vi "project3.vi"() -> ()   [LabVIEW 2020]
uses:
  <vilib>/vision/Image Controls.llb/IMAQ Image.ctl
panel:
  in  "Process":bool
  in  "Stop acquisition":bool
  in  "Acquire":bool
  out "Image":T1(plugin-control)
  in  "Stop program":bool
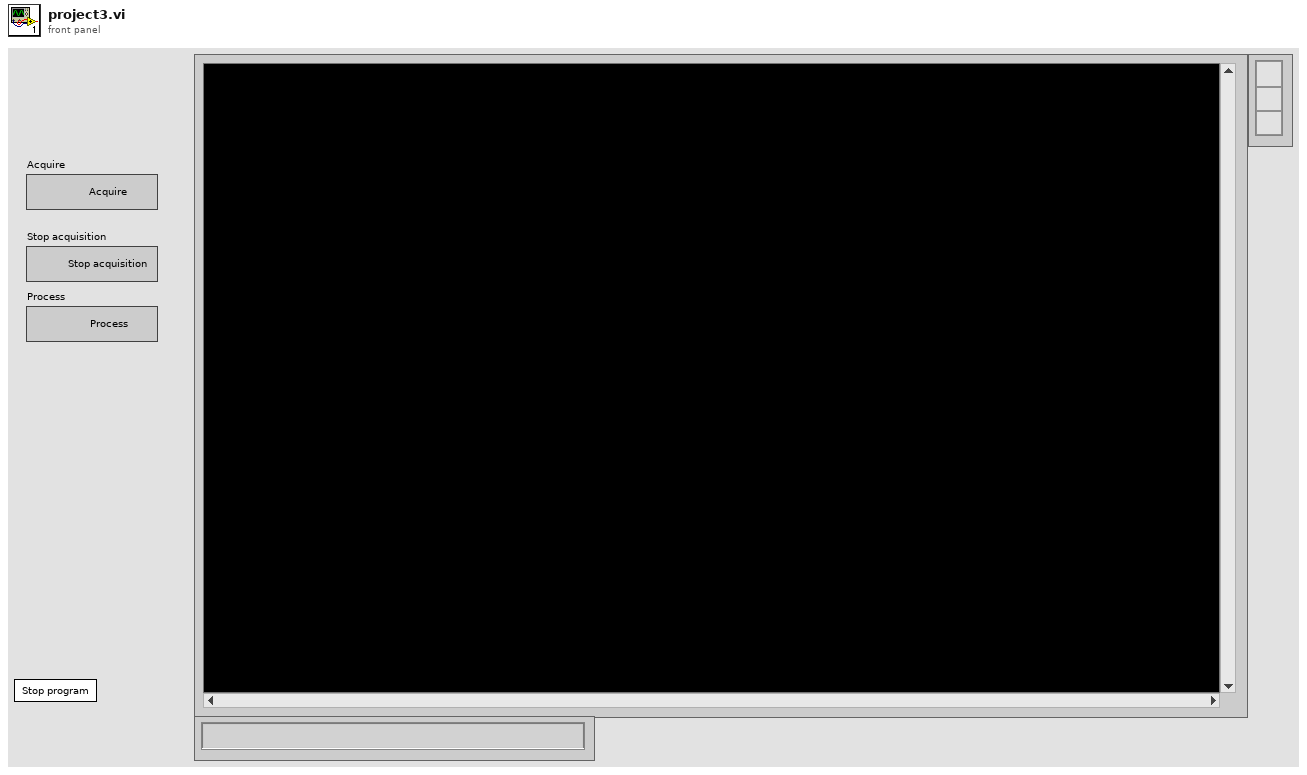
[diagram p1: front panel]
types:
  T1 = typedef "IMAQ Image.ctl" = refnum<image>
  T2 = enum32{"Invalid", "Standard", "Closed", "Hidden", "Minimized", "Maximized"}
  T3 = enum32{"invalid app kind", "Development System", "Run Time System", "Student Edition", "Embedded LabVIEW", "Evaluation", "Custom"}
  T4 = cluster{"Core":cluster{"Current VI Reference":refnum<vi>, "Close Panel on Exit?":bool}, "Aborted":bool, "New Image":T1, "Processing":bool}
  T5 = cluster{"Current VI Reference":refnum<vi>, "Close Panel on Exit?":bool}
  T6 = typedef "Image Type" = u32
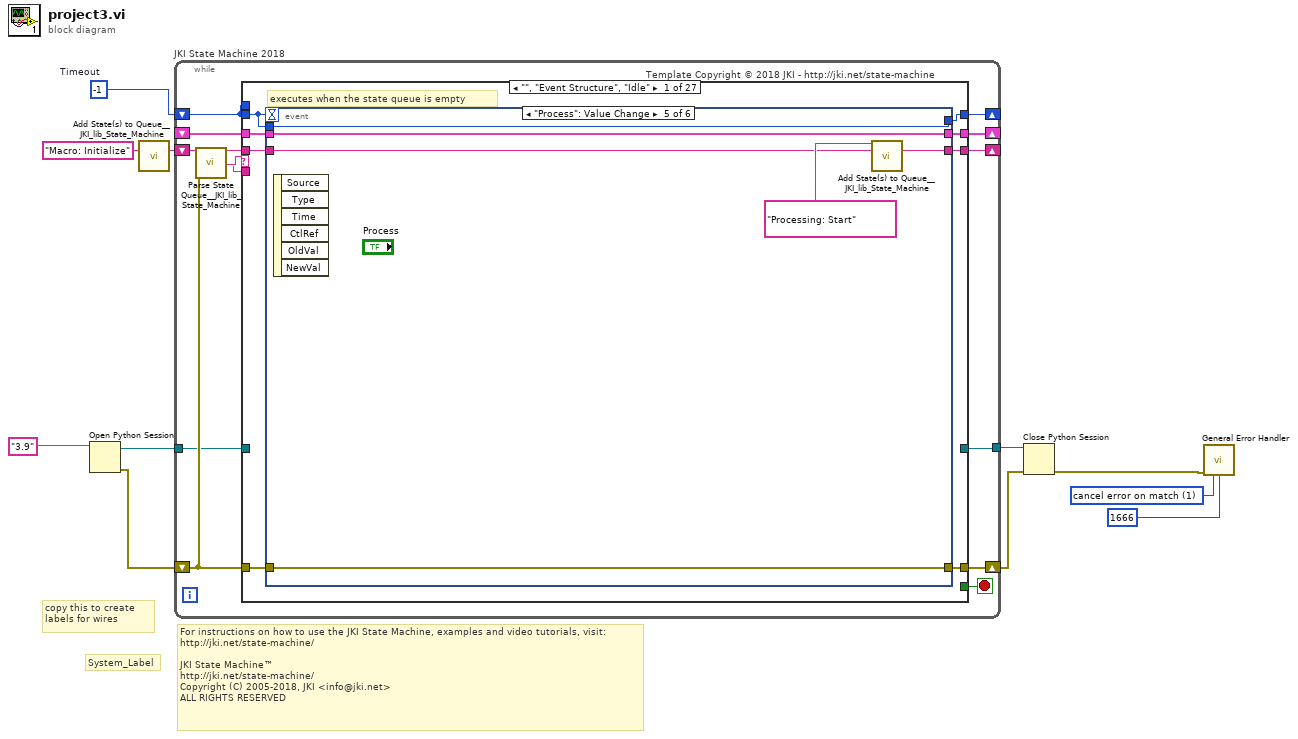
[diagram p0: block diagram]
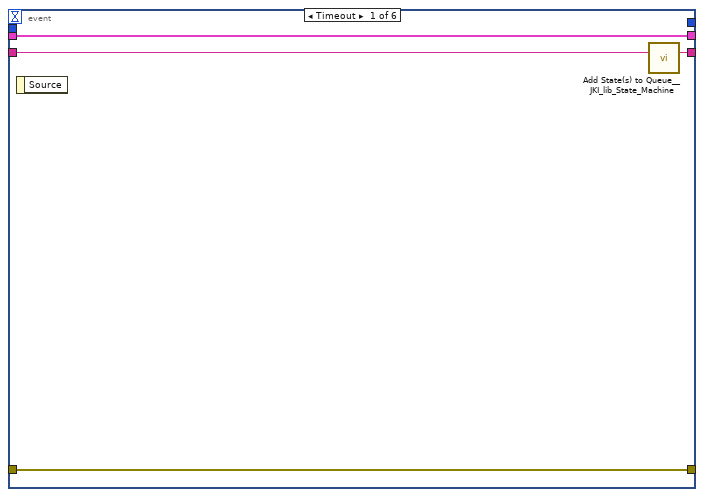
[diagram p2: hidden frame]
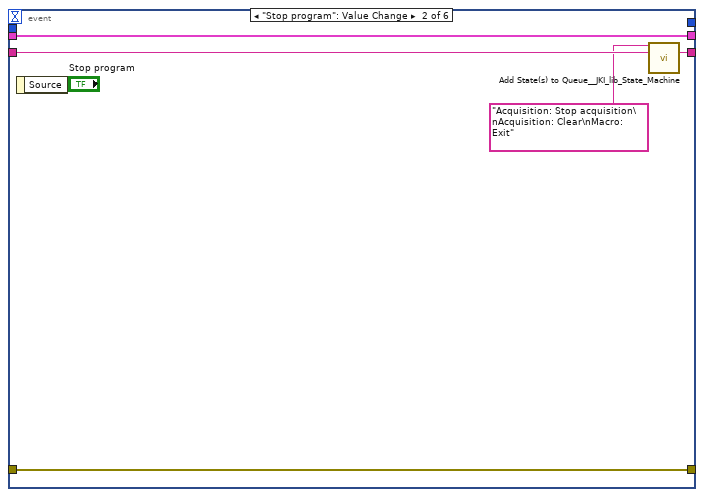
[diagram p3: hidden frame]
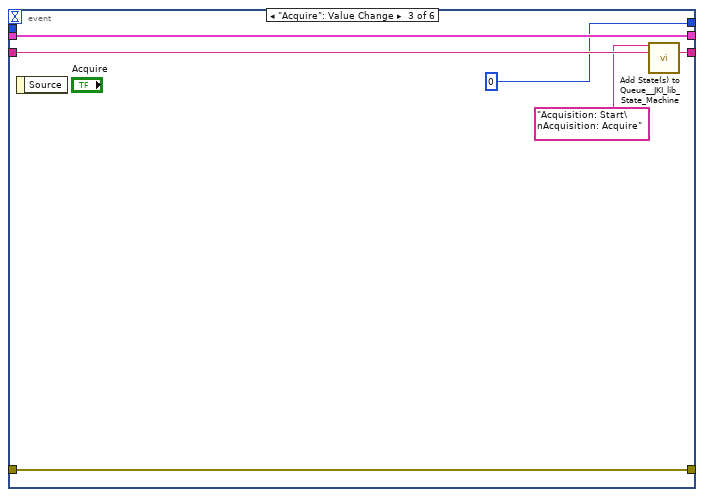
[diagram p4: hidden frame]
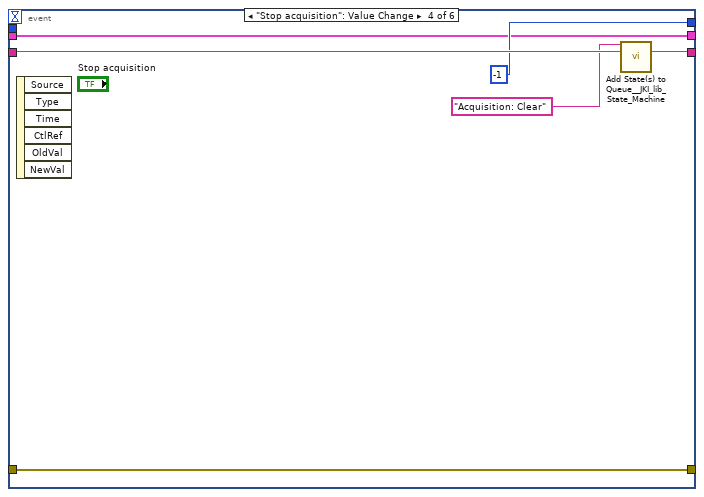
[diagram p5: hidden frame]
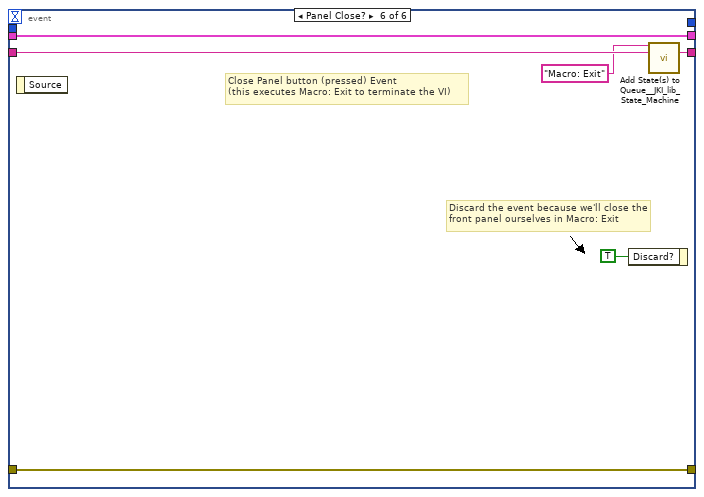
[diagram p6: hidden frame]
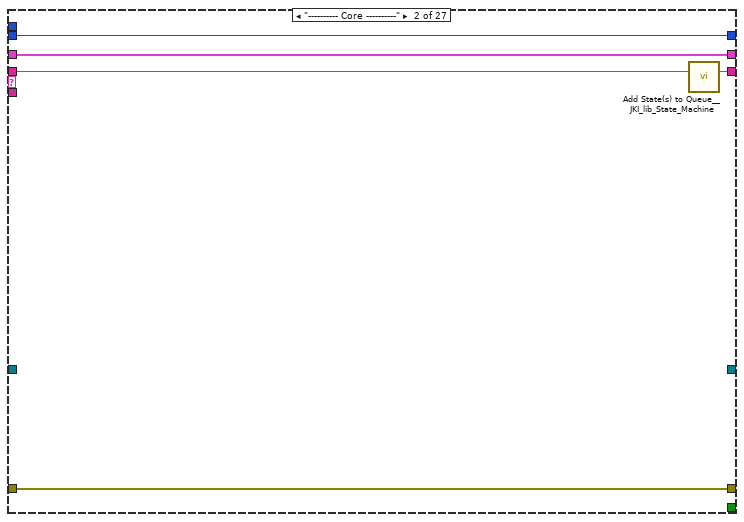
[diagram p7: hidden frame]
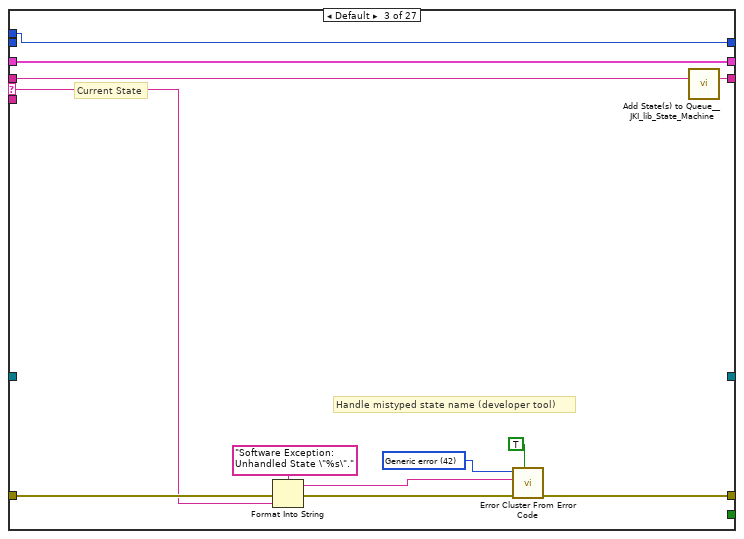
[diagram p8: hidden frame]
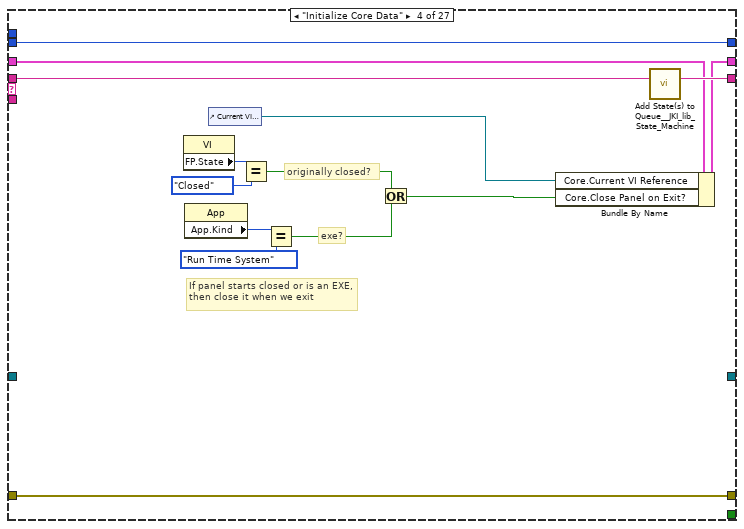
[diagram p9: hidden frame]
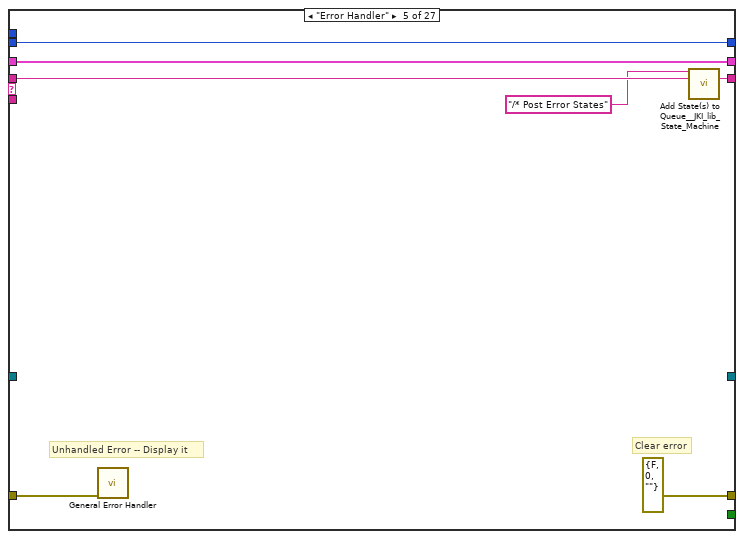
[diagram p10: hidden frame]
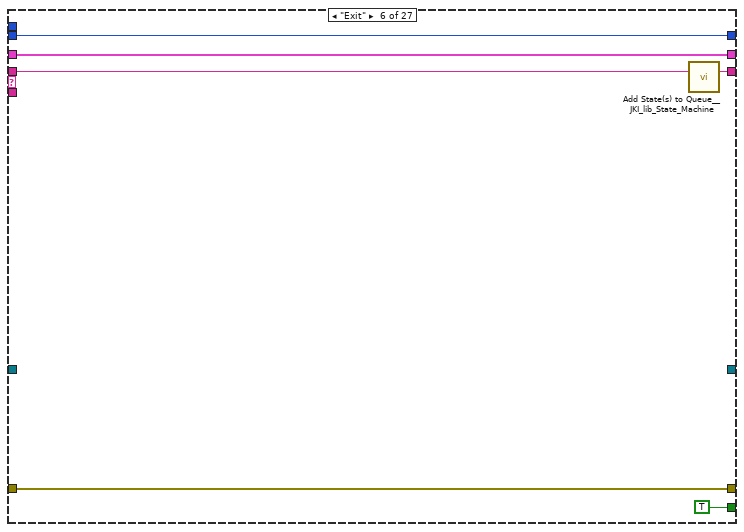
[diagram p11: hidden frame]
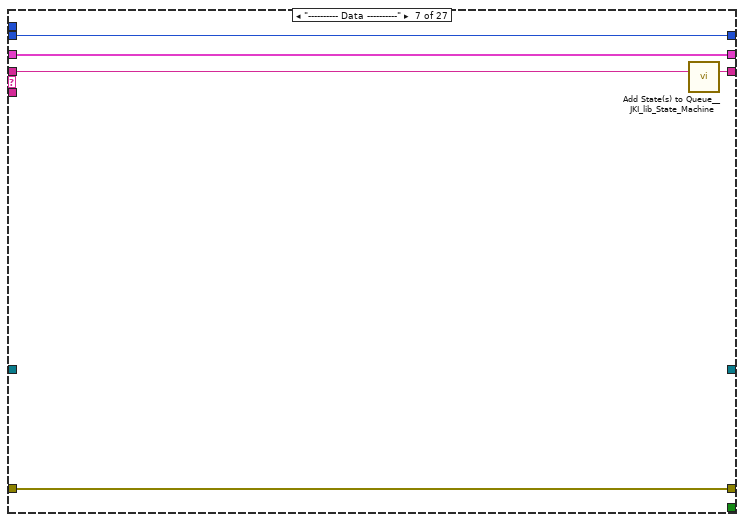
[diagram p12: hidden frame]
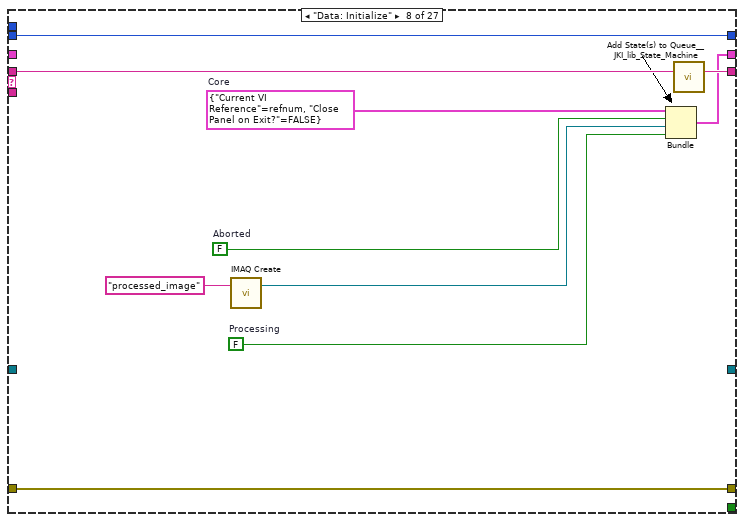
[diagram p13: hidden frame]
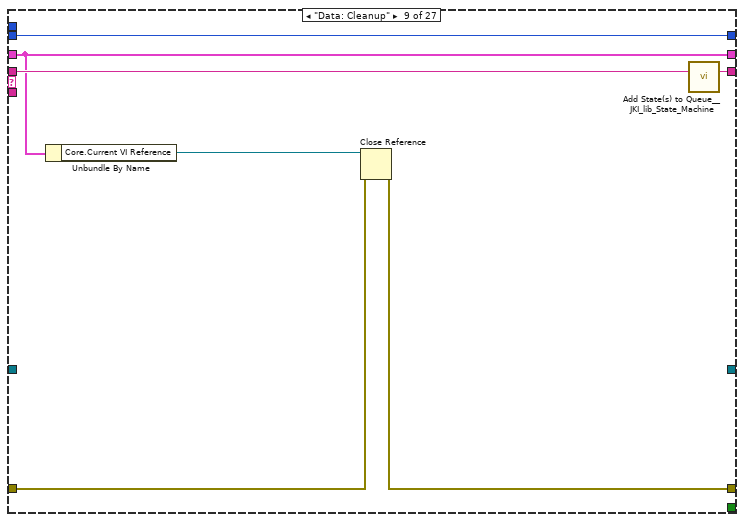
[diagram p14: hidden frame]
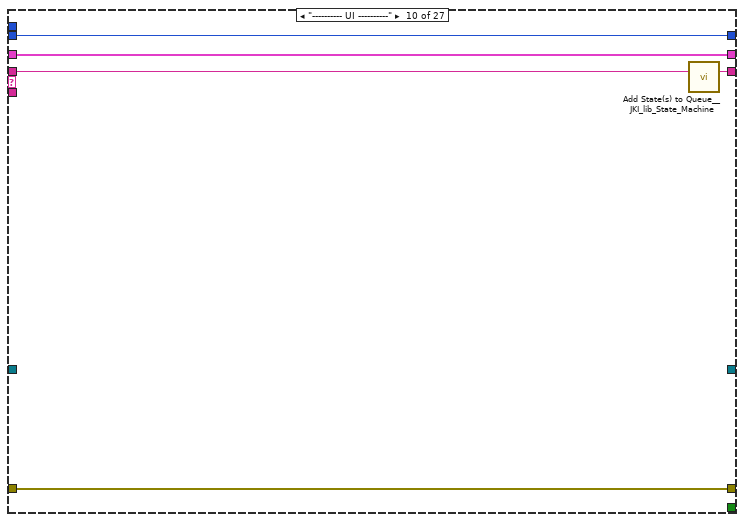
[diagram p15: hidden frame]
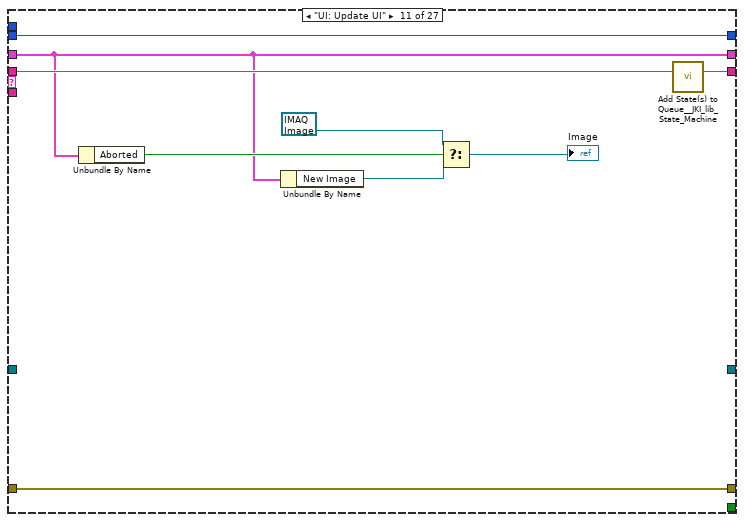
[diagram p16: hidden frame]
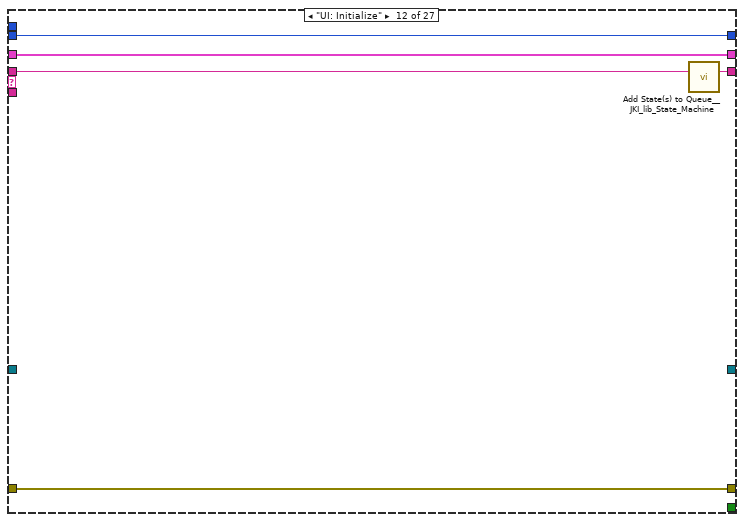
[diagram p17: hidden frame]
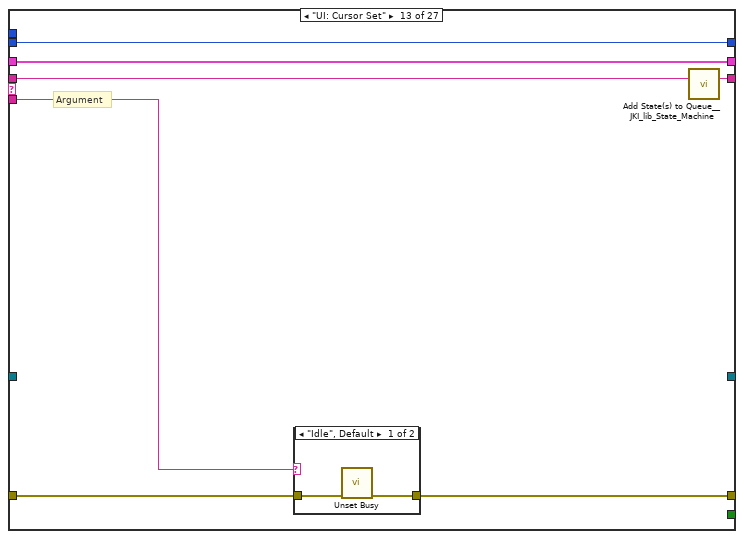
[diagram p18: hidden frame]
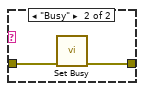
[diagram p19: hidden frame]
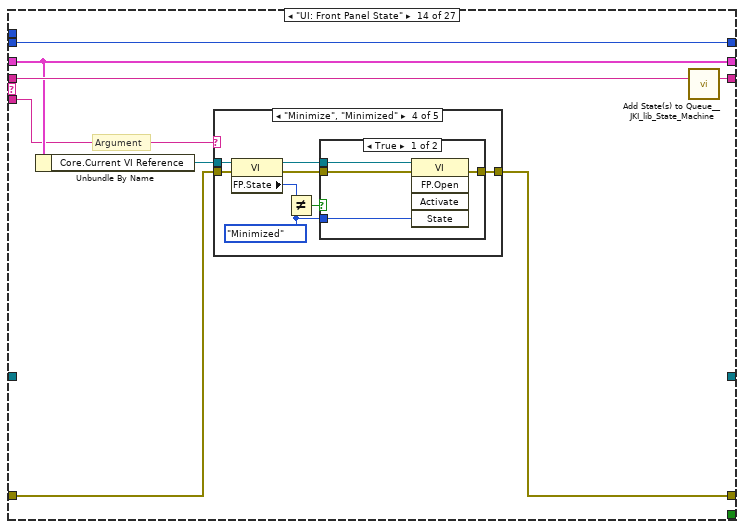
[diagram p20: hidden frame]
diagram:
  w3 = 1 items=["no exception", "cancel error on match", "set error on match"] ("[exception action] (none:0)")
  w9 = -1  # Timeout
  # "For instructions on how to use the JKI State Machine, examples and video tutorials, visit:\nhttp://jki.net/state-machine/\n\nJKI State Machine™\nhttp://jki.net/state-machine/\nCopyright (C) 2005-2018, JKI <info@jki.net>\nALL RIGHTS RESERVED"
  # "copy this to create labels for wires"
  # "System_Label"
  n1 = Open Python Session(python version="3.9" ("Python version")) -> (session out=w8:refnum<k35>, error out=w6:errorcluster)  [unwired: 2 in]
  n2 = call <vilib>:"Add State(s) to Queue__JKI_lib_State_Machine.vi"("State(s) in (\"\")"="Macro: Initialize") -> ("States Out"=w11:string)  [unwired: 14 in]
  n3 = while "JKI State Machine 2018" {
    shift-right: [w18] -> _
    shift-left: _ -> [w17]
    shift-right: [w21] -> w4
    shift-left: w6 -> [w16]
    shift-right: [w20] -> _
    shift-left: w11 -> [w22]
    shift-right: [w15] -> _
    shift-left: w9 -> [w14]
    tunnel: w8 -> [w13]
    tunnel: [w12] -> w5
    stop <- w19 stop-if-true
    # "Template Copyright © 2018 JKI - http://jki.net/state-machine"
    n4 = call <vilib>:"Parse State Queue__JKI_lib_State_Machine.vi"("State Queue"=w22, "Error In (no error)"=w16) -> ("Remaining States"=w24:string, "Current State"=w25:string, "Arguments"=w23:string)  [unwired: 11 in]
    n5 = case shown="\"\", \"Event Structure\", \"Idle\"" w25 {
      selector: w25 -> [_ _ w73 _ _ _ _ _ _ _ _ _ _ _ _ _ _ _ _ _ _ _ _ _ _ _ _]
      tunnel: w24 -> [w33 w71 w77 w97 w104 w110 w115 w125 w132 w137 w145 w151 w158 w170 w240 w246 w257 w262 w269 w286 w293 w302 w307 w312 w319 w339 w344]
      tunnel: w23 -> [_ _ _ _ _ _ _ _ _ _ _ _ w153 w164 _ _ _ _ _ _ _ _ _ _ _ _ _]
      tunnel: w17 -> [w31 w68 w75 w90 w101 w108 w112 _ w127 w134 w141 w149 w156 w166 w237 w243 w254 w259 w264 w284 w289 w298 w304 w309 w315 w335 w341]
      tunnel: [w30 w69 w79 w94 errorcluster {"status"=FALSE, "code"=0, "source"=""} ("error out") w107 w113 w122 w128 w135 w139 w148 w154 w167 w238 w244 w255 w260 w267 w274 w291 w300 w305 w310 w317 w328 w342] -> w21
      tunnel: w16 -> [w29 w69 w78 w94 w100 w107 w113 w122 w129 w135 w139 w148 w155 w168 w238 w244 w255 w260 w267 w275 w291 w300 w305 w310 w317 w327 w342]
      tunnel: [w32 w70 w76 w96 w103 w109 w114 w124 w131 w136 w146 w150 w157 w169 w239 w245 w256 w261 w268 w285 w292 w301 w306 w311 w318 w338 w343] -> w20
      tunnel: [_ _ _ _ _ TRUE _ _ _ _ _ _ _ _ _ _ _ _ _ _ _ _ _ _ _ _ _] -> w19
      tunnel: [w28 w68 w75 w95 w101 w108 w112 w123 w127 w134 w141 w149 w156 w166 w237 w243 w254 w259 w265 w283 w288 w298 w304 w309 w314 w334 w341] -> w18
      tunnel: w14 -> [w26 w67 _ w84 w98 w105 w111 w117 w126 w133 w138 w147 w152 w163 w236 w241 w247 w258 w263 w276 w290 w299 w303 w308 w316 w337 w340]
      tunnel: [w27 w67 w72 w84 w98 w105 w111 w117 w126 w133 w138 w147 w152 w163 w236 w241 w247 w258 w263 w276 w290 w299 w303 w308 w316 w337 w340] -> w15
      tunnel: w14 -> [_ _ w72 _ _ _ _ _ _ _ _ _ _ _ _ _ _ _ _ _ _ _ _ _ _ _ _]
      tunnel: w13 -> [_ _ _ _ _ _ _ _ _ _ _ _ _ _ _ _ _ _ _ _ _ _ _ _ _ w321 _]
      tunnel: [_ _ _ _ _ _ _ _ _ _ _ _ _ _ _ _ _ _ _ _ _ _ _ _ _ w320 _] -> w12
      frame "", "Event Structure", "Idle" {
        # "executes when the state queue is empty"
        n6 = event shown="[4] \"Process\": Value Change" {
          selector: _ -> [_ _ _ _ _ _]
          dyn-events: _ -> [_ _ _ _ _ _]
          timeout: w26 -> [_ _ _ _ _ _]
          tunnel: w33 -> [w37 w42 w48 w53 w55 w66]
          tunnel: [w36 w41 w47 w54 w59 w65] -> w32
          tunnel: w31 -> [w34 w39 w45 w50 w60 w63]
          tunnel: [w35 w40 w46 w49 w56 w64] -> w30
          tunnel: w29 -> [w35 w40 w46 w49 w56 w64]
          tunnel: [w34 w39 w45 w50 w60 w63] -> w28
          tunnel: [_ _ 0 ("Timeout") -1 ("Timeout") w57 _] -> w27
          tunnel: w26 -> [_ _ _ _ w57 _]
          event Timeout {
            n7 = event-data() -> ()  [unwired: 1 in, 1 out]
            n8 = call <vilib>:"Add State(s) to Queue__JKI_lib_State_Machine.vi"("State(s) in (\"\")"=w37) -> ("States Out"=w36:string)  [unwired: 14 in]
          }
          event "Stop program": Value Change {
            n9 = event-data() -> ()  [unwired: 1 in, 1 out]
            n10 = call <vilib>:"Add State(s) to Queue__JKI_lib_State_Machine.vi"("State(s) in Front (\"\")"="Acquisition: Stop acquisition\nAcquisition: Clear\nMacro: Exit", "State(s) in (\"\")"=w42) -> ("States Out"=w41:string)  [unwired: 13 in]
          }
          event "Acquire": Value Change {
            n11 = event-data() -> ()  [unwired: 1 in, 1 out]
            n12 = call <vilib>:"Add State(s) to Queue__JKI_lib_State_Machine.vi"("State(s) in Front (\"\")"="Acquisition: Start\nAcquisition: Acquire", "State(s) in (\"\")"=w48) -> ("States Out"=w47:string)  [unwired: 13 in]
          }
          event "Stop acquisition": Value Change {
            n13 = event-data() -> ()  [unwired: 1 in, 6 out]
            n14 = call <vilib>:"Add State(s) to Queue__JKI_lib_State_Machine.vi"("State(s) in Front (\"\")"="Acquisition: Clear" ("State(s) in Front (\"\")"), "State(s) in (\"\")"=w53) -> ("States Out"=w54:string)  [unwired: 13 in]
          }
          event "Process": Value Change {
            n15 = event-data() -> ()  [unwired: 1 in, 6 out]
            n16 = call <vilib>:"Add State(s) to Queue__JKI_lib_State_Machine.vi"("State(s) in Front (\"\")"="Processing: Start" ("State(s) in Front (\"\")"), "State(s) in (\"\")"=w55) -> ("States Out"=w59:string)  [unwired: 13 in]
          }
          event Panel Close? {
            # "Discard the event because we'll close the front panel ourselves in Macro: Exit"
            # "Close Panel button (pressed) Event\n(this executes Macro: Exit to terminate the VI)"
            n17 = event-data() -> ()  [unwired: 1 in, 1 out]
            n18 = event-data("Discard?"=TRUE) -> ()  [unwired: 1 in, 1 out]
            n19 = call <vilib>:"Add State(s) to Queue__JKI_lib_State_Machine.vi"("State(s) in Front (\"\")"="Macro: Exit", "State(s) in (\"\")"=w66) -> ("States Out"=w65:string)  [unwired: 13 in]
          }
        }
      }
      frame "---------- Core ----------" {
        n20 = call <vilib>:"Add State(s) to Queue__JKI_lib_State_Machine.vi"("State(s) in (\"\")"=w71) -> ("States Out"=w70:string)  [unwired: 14 in]
      }
      frame Default {
        w82 = 42 items=["No error", "Argument error", "Memory is full", "Out of zone", "End of file", "File already open", "Generic file I/O error", "File not found", "File permission error", "Disk is full", "Duplicate path", "Too many files open", "System feature not enabled", "Resource file not found", "Cannot add resource", "Resource not found", "Image not found", "Image memory error", "Pen does not exist", "Config type invalid", "Config token not found", "Config parse error", "Config memory error", "Bad external code format", "Bad external code offset", "External code not present", "Null window", "Destroy window error", "Null menu", "Print aborted", "Bad print record", "Print driver error", "Windows error during printing", "Memory error during printing", "Print dialog error", "Generic print error", "Invalid device refnum", "Device not found", "Device parameter error", "Device unit error", "Cannot open device", "Device call aborted", "Generic error", "Cancelled by user", "Object ID too low", "Object ID too high", "Object not in heap", "Unknown heap", "Unknown object (invalid DefProc)", "Unknown object (DefProc not in table)", "Message out of range", "Invalid (null) method", "Unknown message", "Manager call not supported", "Bad address", "Network operation in progress", "Network operation timed out", "Connection is busy", "Network attribute not supported", "Network error", "Address in use", "System out of memory", "Connection aborted", "Connection refused", "Not connected", "Already connected", "Connection closed", "Initialization error (interapplication manager)", "Bad occurrence", "Wait on unbound occurrence handler", "Occurrence queue overflow", "Datalog type conflict", "Unused", "Unrecognized type (interapplication manager)", "Memory corrupt", "Failed to make temporary DLL", "Old CIN version", "Drag socket not found", "Failed to load drop-object", "Failed to register OLE object", "Failed to release OLE object", "Format specifier type mismatch", "Unknown format specifier", "Too few format specifiers", "Too many format specifiers", "Scan failed", "Newer CIN version", "Error converting to variant", "Runtime menu error", "Password tampered", "Variant attribute not found", "Incompatible variant data type", "Event data is not available", "Event Store is not present", "Occurrence is not found", "Event Queue is not created", "Event info is not available", "Refnum passed is NULL", "Error retrieving Class GUID", "Error retrieving CoClass GUID", "Error retrieving TypeLib GUID.", "Bad built application magic bytes.", "Specific driver is different from the specific driver associated with the Logical Name.", "There is no session opened to the class driver.", "Max Error", "MAX - Error with config objects", "MAX - Error loading configuration", "MAX - Group not supported"]
        # "Current State"
        # "Handle mistyped state name (developer tool)"
        n21 = Format Into String(format string="Software Exception: Unhandled State \"%s\"." ("message"), error in=w78, w73) -> (resulting string=w81:string, error out=w80:errorcluster)  [unwired: 1 in]
        n22 = call <vilib>:"Error Cluster From Error Code.vi"("show call chain? (False)"=TRUE, "error in (no error)"=w80, "error message (\"\")"=w81, "error code (0)"=w82) -> ("error out"=w79:errorcluster)  [unwired: 5 in]
        n23 = call <vilib>:"Add State(s) to Queue__JKI_lib_State_Machine.vi"("State(s) in (\"\")"=w77) -> ("States Out"=w76:string)  [unwired: 14 in]
      }
      frame "Initialize Core Data" {
        # "originally closed?"
        # "exe?"
        # "If panel starts closed or is an EXE, then close it when we exit"
        n24 = property class="VI"() -> ("FP.State"=w87:T2)  [unwired: 2 in, 2 out]
        n25 = property class="App"() -> ("App.Kind"=w93:T3)  [unwired: 2 in, 2 out]
        n26 = control-ref of="Current VI Reference"() -> (w88:refnum<vi>)
        n27 = Equal?(x=w87, y=T2."Closed" ("Front Panel Window:State")) -> (x = y?=w85:bool)
        n28 = Equal?(x=w93, y=T3."Run Time System" ("Application:Kind")) -> (x = y?=w91:bool)
        n29 = Or(x=w85, y=w91) -> (x .or. y?=w89:bool)
        n30 = Bundle By Name(cluster=w90, "Core.Current VI Reference"=w88, "Core.Close Panel on Exit?"=w89) -> (w95:T4)
        n31 = call <vilib>:"Add State(s) to Queue__JKI_lib_State_Machine.vi"("State(s) in (\"\")"=w97) -> ("States Out"=w96:string)  [unwired: 14 in]
      }
      frame "Error Handler" {
        # "Unhandled Error -- Display it"
        # "Clear error"
        n32 = call <vilib>:"General Error Handler.vi"("error in (no error)"=w100) -> ()  [unwired: 10 in, 5 out]
        n33 = call <vilib>:"Add State(s) to Queue__JKI_lib_State_Machine.vi"("State(s) in Front (\"\")"="/* Post Error States", "State(s) in (\"\")"=w104) -> ("States Out"=w103:string)  [unwired: 13 in]
      }
      frame "Exit" {
        n34 = call <vilib>:"Add State(s) to Queue__JKI_lib_State_Machine.vi"("State(s) in (\"\")"=w110) -> ("States Out"=w109:string)  [unwired: 14 in]
      }
      frame "---------- Data ----------" {
        n35 = call <vilib>:"Add State(s) to Queue__JKI_lib_State_Machine.vi"("State(s) in (\"\")"=w115) -> ("States Out"=w114:string)  [unwired: 14 in]
      }
      frame "Data: Initialize" {
        w116 = FALSE  # Processing
        w120 = T5 {"Current VI Reference"=refnum, "Close Panel on Exit?"=FALSE}  # Core
        w121 = FALSE  # Aborted
        n36 = call "IMAQ Create"("Image Name"="processed_image") -> ("New Image"=w119:T1)  [unwired: 4 in, 1 out]
        n37 = Bundle("Core"=w120, "Aborted"=w121, "New Image"=w119, "Processing"=w116) -> (w123:T4)  [unwired: 1 in]
        n38 = call <vilib>:"Add State(s) to Queue__JKI_lib_State_Machine.vi"("State(s) in (\"\")"=w125) -> ("States Out"=w124:string)  [unwired: 14 in]
      }
      frame "Data: Cleanup" {
        n39 = Unbundle By Name(w127) -> ("Core.Current VI Reference"=w130:refnum<vi>)
        n40 = Close Reference(reference=w130, error in (no error)=w129) -> (error out=w128:errorcluster)
        n41 = call <vilib>:"Add State(s) to Queue__JKI_lib_State_Machine.vi"("State(s) in (\"\")"=w132) -> ("States Out"=w131:string)  [unwired: 14 in]
      }
      frame "---------- UI ----------" {
        n42 = call <vilib>:"Add State(s) to Queue__JKI_lib_State_Machine.vi"("State(s) in (\"\")"=w137) -> ("States Out"=w136:string)  [unwired: 14 in]
      }
      frame "UI: Update UI" {
        n43 = Unbundle By Name(w141) -> ("Aborted"=w144:bool)
        n44 = Unbundle By Name(w141) -> ("New Image"=w142:T1)
        n45 = Select(t=T1 refnum, s=w144, f=w142) -> (s? t:f=→"Image":T1)
        n46 = call <vilib>:"Add State(s) to Queue__JKI_lib_State_Machine.vi"("State(s) in (\"\")"=w145) -> ("States Out"=w146:string)  [unwired: 14 in]
      }
      frame "UI: Initialize" {
        n47 = call <vilib>:"Add State(s) to Queue__JKI_lib_State_Machine.vi"("State(s) in (\"\")"=w151) -> ("States Out"=w150:string)  [unwired: 14 in]
      }
      frame "UI: Cursor Set" {
        # "Argument"
        n48 = case shown="\"Idle\", Default" w153 {
          tunnel: w155 -> [w160 w162]
          tunnel: [w159 w161] -> w154
          frame "Idle", Default {
            n49 = call <vilib>:"Unset Busy.vi"("error in (no error)"=w160) -> ("error out"=w159:errorcluster)  [unwired: 10 in]
          }
          frame "Busy" {
            n50 = call <vilib>:"Set Busy.vi"("error in (no error)"=w162) -> ("error out"=w161:errorcluster)  [unwired: 9 in, 1 out]
          }
        }
        n51 = call <vilib>:"Add State(s) to Queue__JKI_lib_State_Machine.vi"("State(s) in (\"\")"=w158) -> ("States Out"=w157:string)  [unwired: 14 in]
      }
      frame "UI: Front Panel State" {
        # "Argument"
        n52 = Unbundle By Name(w166) -> ("Core.Current VI Reference"=w165:refnum<vi>)
        n53 = case shown="\"Minimize\", \"Minimized\"" w164 {
          tunnel: w168 -> [w176 w191 w202 w215 w228]
          tunnel: [w178 w192 w204 w217 w230] -> w167
          tunnel: w165 -> [w177 w189 w203 w216 w229]
          frame "Open", "Standard", Default {
            w171 = T2."Standard" ("State")
            n54 = property class="VI"(reference=w177, error in=w176) -> (reference out=w174:refnum<vi>, error out=w175:errorcluster, "FP.State"=w173:T2)
            n55 = Not Equal?(x=w173, y=w171) -> (x != y?=w172:bool)
            n56 = case shown="True" w172 {
              tunnel: [w182 w184] -> w178
              tunnel: w175 -> [w181 w184]
              tunnel: w174 -> [w180 _]
              tunnel: w171 -> [w179 _]
              frame True {
                n57 = invoke class="VI" method="FP.Open"(reference=w180, error in=w181, "Activate"=TRUE, "State"=w179) -> (error out=w182:errorcluster)  [unwired: 1 in, 4 out]
              }
              frame False {
              }
            }
          }
          frame "Close", "Closed" {
            n58 = property class="VI"(reference=w189, error in=w191) -> (reference out=w188:refnum<vi>, error out=w190:errorcluster, "FP.State"=w186:T2)
            n59 = Not Equal?(x=w186, y=T2."Closed" ("Front Panel Window:State")) -> (x != y?=w185:bool)
            n60 = case shown="True" w185 {
              tunnel: [w193 w196] -> w192
              tunnel: w190 -> [w193 w195]
              tunnel: w188 -> [_ w194]
              frame False {
              }
              frame True {
                n61 = invoke class="VI" method="FP.Close"(reference=w194, error in=w195) -> (error out=w196:errorcluster)  [unwired: 1 in, 2 out]
              }
            }
          }
          frame "Hidden", "Hide" {
            w197 = T2."Hidden" ("State")
            n62 = property class="VI"(reference=w203, error in=w202) -> (reference out=w200:refnum<vi>, error out=w201:errorcluster, "FP.State"=w199:T2)
            n63 = Not Equal?(x=w199, y=w197) -> (x != y?=w198:bool)
            n64 = case shown="True" w198 {
              tunnel: [w208 w209] -> w204
              tunnel: w201 -> [w207 w209]
              tunnel: w200 -> [w206 _]
              tunnel: w197 -> [w205 _]
              frame True {
                n65 = invoke class="VI" method="FP.Open"(reference=w206, error in=w207, "State"=w205) -> (error out=w208:errorcluster)  [unwired: 2 in, 4 out]
              }
              frame False {
              }
            }
          }
          frame "Minimize", "Minimized" {
            w210 = T2."Minimized" ("State")
            n66 = property class="VI"(reference=w216, error in=w215) -> (reference out=w213:refnum<vi>, error out=w214:errorcluster, "FP.State"=w212:T2)
            n67 = Not Equal?(x=w212, y=w210) -> (x != y?=w211:bool)
            n68 = case shown="True" w211 {
              tunnel: [w221 w222] -> w217
              tunnel: w214 -> [w220 w222]
              tunnel: w213 -> [w219 _]
              tunnel: w210 -> [w218 _]
              frame True {
                n69 = invoke class="VI" method="FP.Open"(reference=w219, error in=w220, "State"=w218) -> (error out=w221:errorcluster)  [unwired: 2 in, 4 out]
              }
              frame False {
              }
            }
          }
          frame "Maximize", "Maximized" {
            w223 = T2."Maximized" ("State")
            n70 = property class="VI"(reference=w229, error in=w228) -> (reference out=w226:refnum<vi>, error out=w227:errorcluster, "FP.State"=w225:T2)
            n71 = Not Equal?(x=w225, y=w223) -> (x != y?=w224:bool)
            n72 = case shown="True" w224 {
              tunnel: [w234 w235] -> w230
              tunnel: w227 -> [w233 w235]
              tunnel: w226 -> [w232 _]
              tunnel: w223 -> [w231 _]
              frame True {
                n73 = invoke class="VI" method="FP.Open"(reference=w232, error in=w233, "State"=w231) -> (error out=w234:errorcluster)  [unwired: 2 in, 4 out]
              }
              frame False {
              }
            }
          }
        }
        n74 = call <vilib>:"Add State(s) to Queue__JKI_lib_State_Machine.vi"("State(s) in (\"\")"=w170) -> ("States Out"=w169:string)  [unwired: 14 in]
      }
      frame "---------- Macro ----------" {
        n75 = call <vilib>:"Add State(s) to Queue__JKI_lib_State_Machine.vi"("State(s) in (\"\")"=w240) -> ("States Out"=w239:string)  [unwired: 14 in]
      }
      frame "Macro: Initialize" {
        w242 = "Data: Initialize\nInitialize Core Data\nUI: Initialize\nUI: Front Panel State >> Open"  # Data: Initialize Initialize Core Data UI: Initialize UI: Front Panel State >> Open
        n76 = call <vilib>:"Add State(s) to Queue__JKI_lib_State_Machine.vi"("State(s) in Front (\"\")"=w242, "State(s) in (\"\")"=w246) -> ("States Out"=w245:string)  [unwired: 13 in]
      }
      frame "Macro: Exit" {
        n77 = Unbundle By Name(w254) -> ("Core.Close Panel on Exit?"=w253:bool)
        n78 = Select(t="UI: Front Panel State >> Close", s=w253, f="") -> (s? t:f=w250:string)
        n79 = call <vilib>:"Add State(s) to Queue__JKI_lib_State_Machine.vi"("State(s) in (\"\")"=w250, "State(s) at Back (\"\")"="Data: Cleanup\nExit") -> ("States Out"=w248:string)  [unwired: 13 in]
        n80 = call <vilib>:"Add State(s) to Queue__JKI_lib_State_Machine.vi"("State(s) in Front (\"\")"=w248, "State(s) in (\"\")"=w257) -> ("States Out"=w256:string)  [unwired: 13 in]
      }
      frame "---------- Acquisition ----------" {
        n81 = call <vilib>:"Add State(s) to Queue__JKI_lib_State_Machine.vi"("State(s) in (\"\")"=w262) -> ("States Out"=w261:string)  [unwired: 14 in]
      }
      frame "Acquisition: Start" {
        n82 = Bundle By Name(cluster=w264, "Aborted"=FALSE) -> (w265:T4)
        n83 = call <vilib>:"Add State(s) to Queue__JKI_lib_State_Machine.vi"("State(s) in (\"\")"=w269) -> ("States Out"=w268:string)  [unwired: 14 in]
      }
      frame "Acquisition: Acquire" {
        w271 = "Event Structure \nUI: Update UI\nAcquisition: Acquire"  # Looping States
        w279 = "UI: Update UI"  # Done States
        w281 = T6 5 items=["Grayscale (U8)", "Grayscale (I16)", "Grayscale (SGL)", "Complex (CSG)", "RGB (U32)", "HSL (U32)", "RGB (U64)", "Grayscale (U16)"] ("Image Type")
        n84 = Unbundle By Name(w284) -> ("Aborted"=w280:bool, "Processing"=w272:bool)
        n85 = call "Vision Acquisition"("error in"=w275) -> ("Image Out"=w277:T1, "error out"=w274:errorcluster)  [unwired: 24 in, 1 out]
        n86 = call "IMAQ Cast Image 2"("Image Src"=w277, "Image Type"=w281) -> ("Image Dst Out"=w282:T1)  [unwired: 12 in, 1 out]
        n87 = Bundle By Name(cluster=w284, "New Image"=w282) -> (w283:T4)
        n88 = Select(t="Event Structure \nProcessing: Process\nUI: Update UI\nAcquisition: Acquire", s=w272, f=w271) -> (s? t:f=w273:string)
        n89 = Select(t=w279, s=w280, f=w273) -> (s? t:f=w278:string)
        n90 = call <vilib>:"Add State(s) to Queue__JKI_lib_State_Machine.vi"("State(s) in Front (\"\")"=w278, "State(s) in (\"\")"=w286) -> ("States Out"=w285:string)  [unwired: 13 in]
      }
      frame "Acquisition: Stop acquisition" {
        n91 = Bundle By Name(cluster=w289, "Aborted"=TRUE) -> (w288:T4)
        n92 = call <vilib>:"Add State(s) to Queue__JKI_lib_State_Machine.vi"("State(s) in (\"\")"=w293) -> ("States Out"=w292:string)  [unwired: 14 in]
      }
      frame "Acquisition: Clear" {
        n93 = Unbundle By Name(w298) -> ("Aborted"=w297:bool)
        n94 = Select(t="UI: Update UI", s=w297, f="Acquisition: Stop acquisition") -> (s? t:f=w295:string)
        n95 = call <vilib>:"Add State(s) to Queue__JKI_lib_State_Machine.vi"("State(s) in Front (\"\")"=w295, "State(s) in (\"\")"=w302) -> ("States Out"=w301:string)  [unwired: 13 in]
      }
      frame "Acquisition: OK" {
        n96 = call <vilib>:"Add State(s) to Queue__JKI_lib_State_Machine.vi"("State(s) in (\"\")"=w307) -> ("States Out"=w306:string)  [unwired: 14 in]
      }
      frame "---------- Processing ----------" {
        n97 = call <vilib>:"Add State(s) to Queue__JKI_lib_State_Machine.vi"("State(s) in (\"\")"=w312) -> ("States Out"=w311:string)  [unwired: 14 in]
      }
      frame "Processing: Start" {
        n98 = Bundle By Name(cluster=w315, "Processing"=TRUE ("IsFaceDetectionON")) -> (w314:T4)
        n99 = call <vilib>:"Add State(s) to Queue__JKI_lib_State_Machine.vi"("State(s) in (\"\")"=w319) -> ("States Out"=w318:string)  [unwired: 14 in]
      }
      frame "Processing: Process" {
        n100 = Unbundle By Name(w335) -> ("New Image"=w332:T1)
        n101 = call <vilib>:"Application Directory.vi"() -> ("Application Directory"=w324:path)
        n102 = call "IMAQ ColorImageToArray"("Image"=w332, "error in (no error)"=w327) -> ("Image Pixels (U32)"=w331:u32[][], "error out"=w326:errorcluster)  [unwired: 2 in, 1 out]
        n103 = Build Path(base path=w324, name or relative path="python\\process_image.py") -> (appended path=w323:path)
        n104 = node(w321, w323, "get_image" ("function name"), w326, w331, w331) -> (w320:refnum<k35>, w329:errorcluster, w330:u32[][])  [unwired: 1 in, 2 out]
        n105 = call "IMAQ ArrayToColorImage"("Image Pixels (U32)"=w330, "Image"=w332, "error in (no error)"=w329) -> ("Image Out"=w333:T1, "error out"=w328:errorcluster)  [unwired: 2 in]
        n106 = Bundle By Name(cluster=w335, "New Image"=w333) -> (w334:T4)
        n107 = call <vilib>:"Add State(s) to Queue__JKI_lib_State_Machine.vi"("State(s) in Front (\"\")"="UI: Update UI" ("State(s) in Front (\"\")"), "State(s) in (\"\")"=w339) -> ("States Out"=w338:string)  [unwired: 13 in]
      }
      frame "Processing: Ok" {
        n108 = call <vilib>:"Add State(s) to Queue__JKI_lib_State_Machine.vi"("State(s) in (\"\")"=w344) -> ("States Out"=w343:string)  [unwired: 14 in]
      }
    }
  }
  n109 = Close Python Session(session in=w5, error in=w4) -> (11:w1:errorcluster)
  n110 = call <vilib>:"General Error Handler.vi"("error in (no error)"=w1, "[exception action] (none:0)"=w3, "[exception code]"=1666) -> ()  [unwired: 8 in, 5 out]
